vi "BRig_RT__Case_Exp__State_initTrial__DAB_flipLR.vi"(10 "input_DAB_flipLR_nTrial":u16, 11 "input_nTrial":u16) -> (2 "output_switchedLR":bool, 3 "output_flipOccurred":bool)   [LabVIEW 2014]
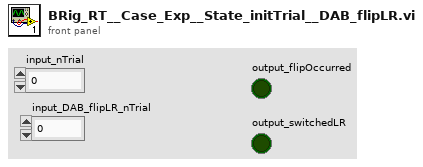
[diagram p1: front panel]
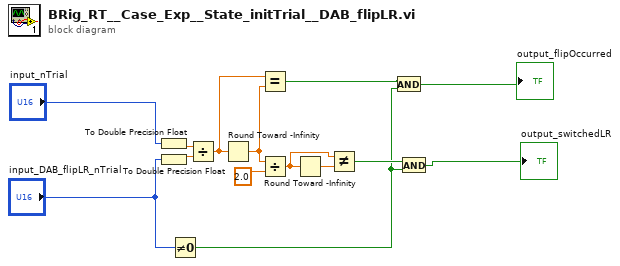
[diagram p0: block diagram]
diagram:
  n1 = To Double Precision Float(number="input_nTrial") -> (double precision float=w14:dbl)
  n2 = To Double Precision Float(number="input_DAB_flipLR_nTrial") -> (double precision float=w13:dbl)
  n3 = Not Equal To 0?(x="input_DAB_flipLR_nTrial") -> (x != 0?=w2:bool)
  n4 = Divide(x=w14, y=w13) -> (x/y=w11:dbl)
  n5 = Round Toward -Infinity(1:w11) -> (0:w10:dbl)
  n6 = Equal?(x=w11, y=w10) -> (x = y?=w5:bool)
  n7 = Divide(x=w10, y=2.0) -> (x/y=w7:dbl)
  n8 = Round Toward -Infinity(1:w7) -> (0:w8:dbl)
  n9 = Not Equal?(x=w7, y=w8) -> (x != y?=w3:bool)
  n10 = And(x=w5, y=w2) -> (x .and. y?=→"output_flipOccurred":bool)
  n11 = And(x=w3, y=w2) -> (x .and. y?=→"output_switchedLR":bool)
